vi "Get Message String.vi"(8 "error in (no error)":errorcluster, 11 "SECS-II Class in":refnum<class "SECS-II Class.lvclass">) -> (0 "error out":errorcluster, 2 "String":string, 3 "SECS-II Class out":refnum<class "SECS-II Class.lvclass">)   [LabVIEW 2020, in "SECS Communication.lvlib" / "SECS-II Class.lvclass"]
uses:
  SECS-II Class.lvclass
  SECS-II Class.lvclass/SECS-II Class.ctl
  Variant To Data_ASCII.vi
  Variant To Data_Character.vi
  Variant To Data_Binary.vi
  Variant To Data_Boolean.vi
  Variant To Data_J.vi
  Variant To Data_I1.vi
  Variant To Data_I2.vi
  Variant To Data_I4.vi
  Variant To Data_I8.vi
  Variant To Data_U1.vi
  Variant To Data_U2.vi
  Variant To Data_U4.vi
  Variant To Data_U8.vi
  Variant To Data_F4.vi
  Variant To Data_F8.vi
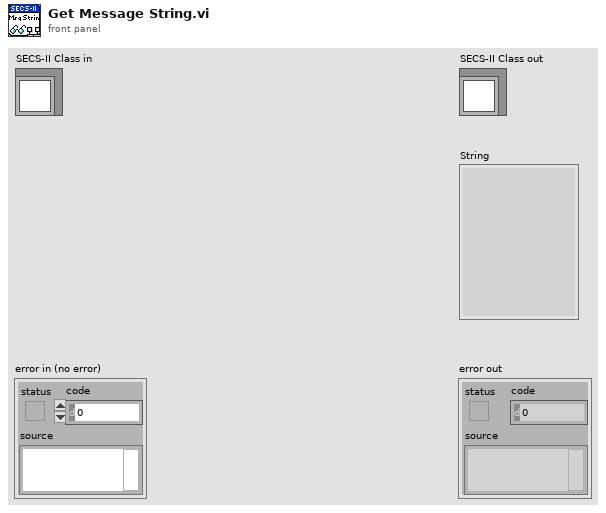
[diagram p1: front panel]
types:
  T1 = typedef "SECS Communication.lvlib/SECS-II Class.lvclass/Message Data.ctl" = cluster{"Index":i32, "Data Item Format":T2, "Format Code":T3, "Parent Index":i32, "Child Index":i32[], "Data":variant}
  T2 = typedef "SECS Communication.lvlib/SECS-II Class.lvclass/Data Item Format.ctl" = enum16{"Data Type", "Value"}
  T3 = typedef "SECS Communication.lvlib/SECS-II Class.lvclass/Format Code.ctl" = enum16{"L", "A", "B", "Boolean", "J", "I1", "I2", "I4", "I8", "U1", "U2", "U4", "U8", "F4", "F8", "Char"}
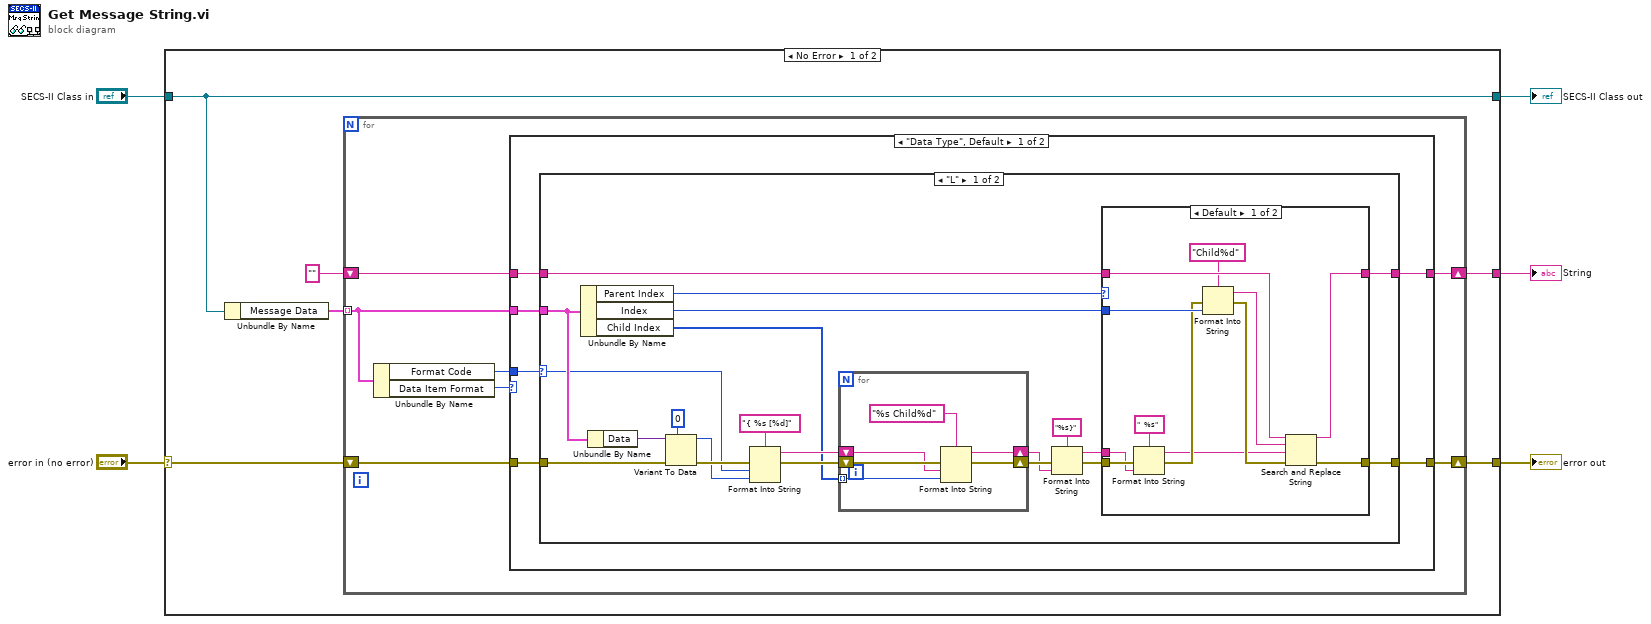
[diagram p0: block diagram]
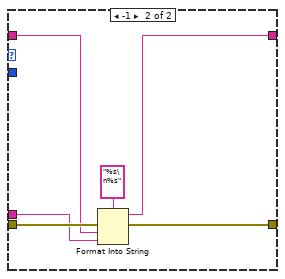
[diagram p2: hidden frame]
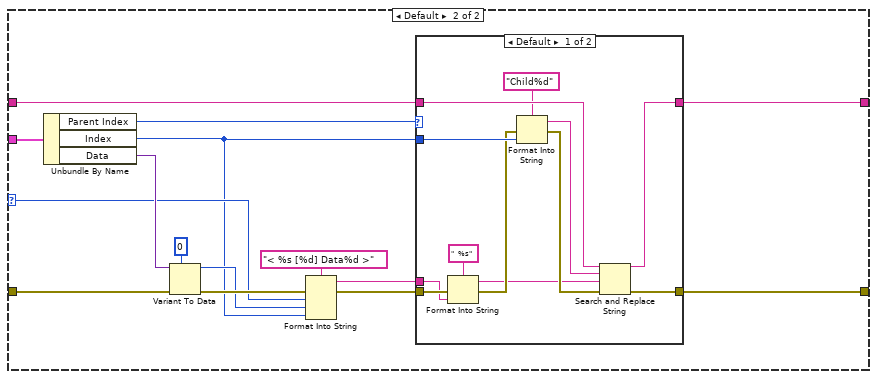
[diagram p3: hidden frame]
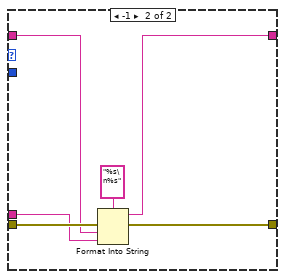
[diagram p4: hidden frame]
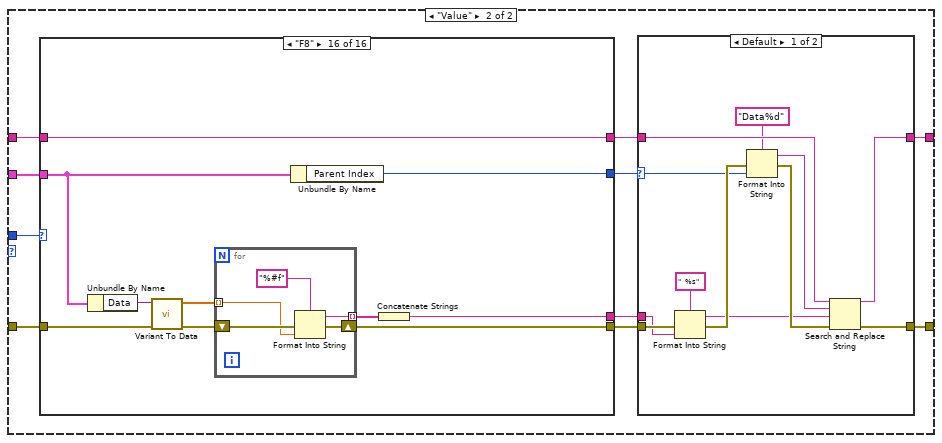
[diagram p5: hidden frame]
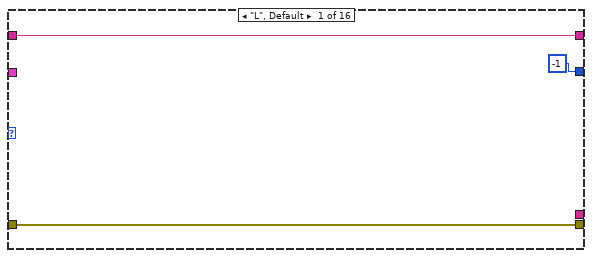
[diagram p7: hidden frame]
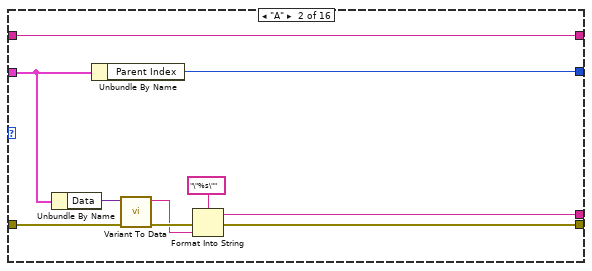
[diagram p8: hidden frame]
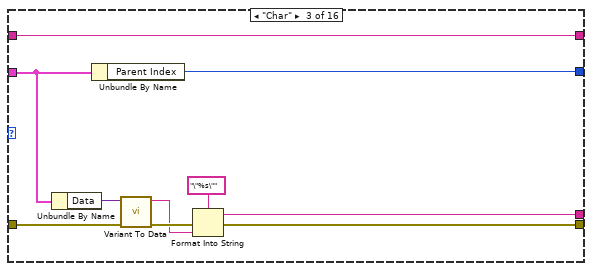
[diagram p9: hidden frame]
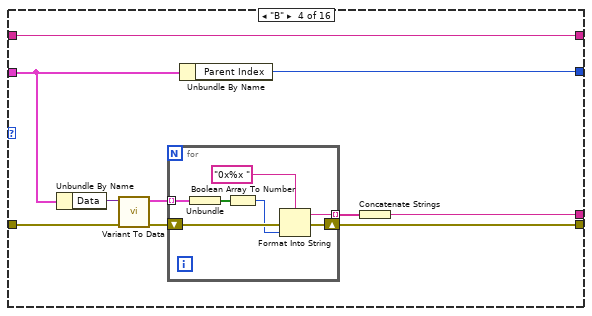
[diagram p10: hidden frame]
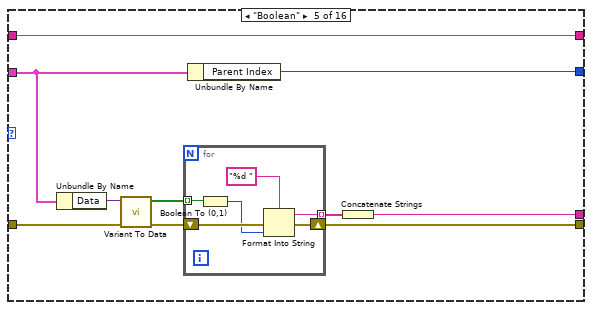
[diagram p11: hidden frame]
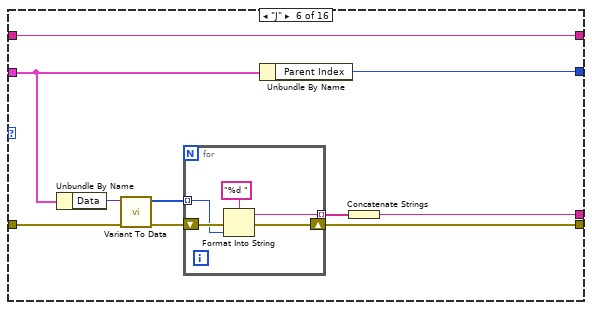
[diagram p12: hidden frame]
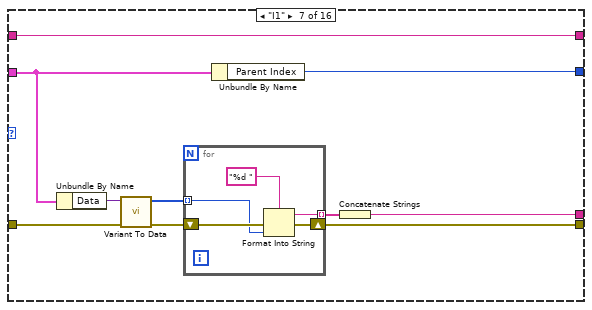
[diagram p13: hidden frame]
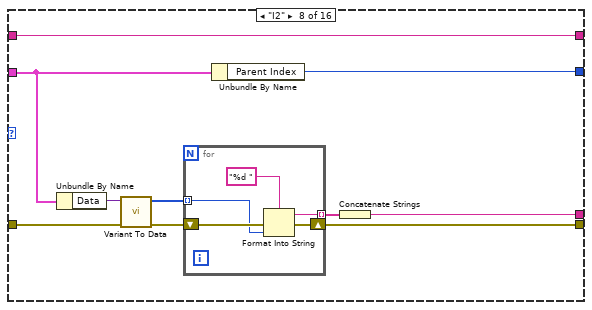
[diagram p14: hidden frame]
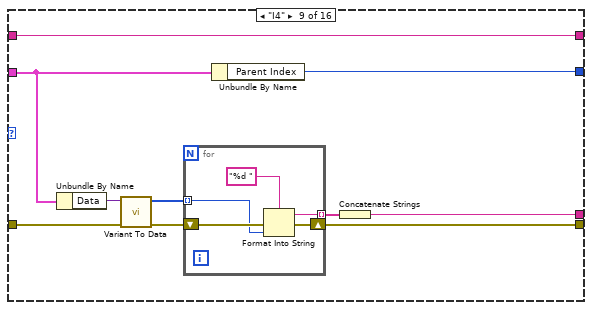
[diagram p15: hidden frame]
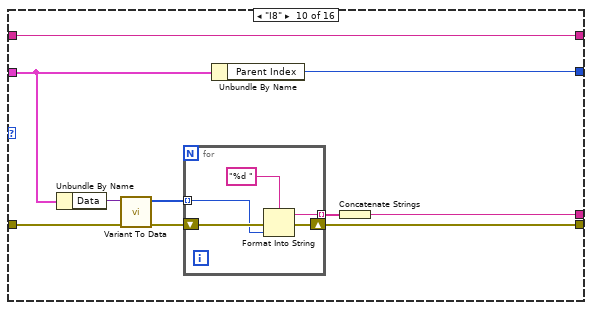
[diagram p16: hidden frame]
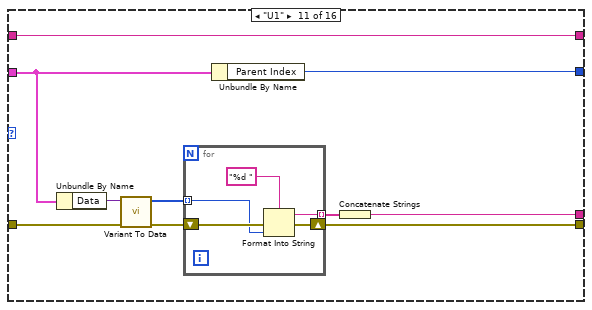
[diagram p17: hidden frame]
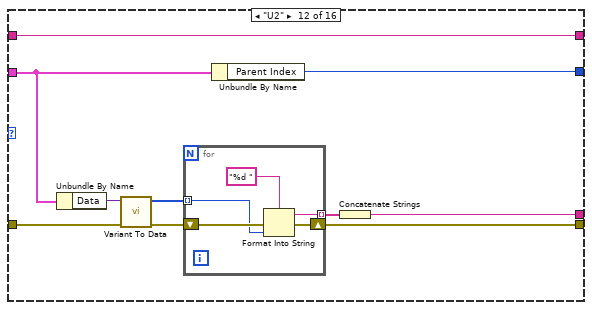
[diagram p18: hidden frame]
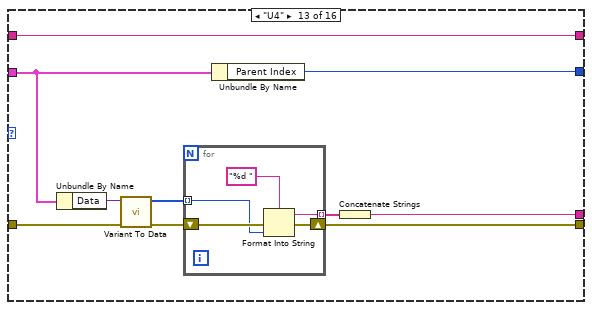
[diagram p19: hidden frame]
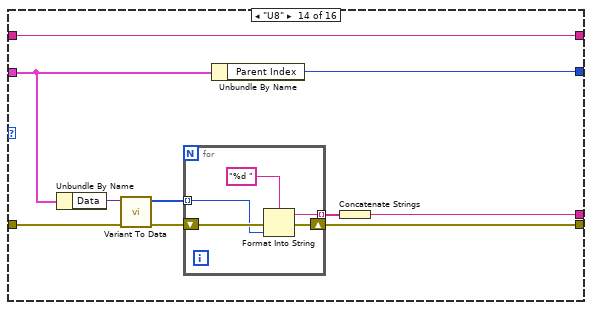
[diagram p20: hidden frame]
diagram:
  n1 = case shown="No Error" "error in (no error)" {
    selector: "error in (no error)" -> [w11 w349]
    tunnel: [w10 w349] -> w5
    tunnel: [w7 w348] -> w4
    tunnel: "SECS-II Class in" -> [w7 w348]
    tunnel: [w6 _] -> w3
    frame No Error {
      n2 = Unbundle By Name(w7) -> ("Message Data"=w8:T1[])
      n3 = for {
        tunnel: w8 -> [w16] mode=indexing
        shift-right: [w12] -> w10
        shift-left: w11 -> [w18]
        shift-right: [w13] -> w6
        shift-left: "" -> [w15]
        n4 = Unbundle By Name(w16) -> ("Format Code"=w14:T3, "Data Item Format"=w17:T2)
        n5 = case shown="\"Data Type\", Default" w17 {
          tunnel: w18 -> [w23 w111]
          tunnel: w16 -> [w22 w109]
          tunnel: w15 -> [w21 w110]
          tunnel: w14 -> [w24 w112]
          tunnel: [w20 w104] -> w13
          tunnel: [w19 w103] -> w12
          frame "Data Type", Default {
            n6 = case shown="\"L\"" w24 {
              selector: w24 -> [w25 w78]
              tunnel: w23 -> [w45 w82]
              tunnel: w22 -> [w37 w84]
              tunnel: w21 -> [w36 w76]
              tunnel: [w34 w71] -> w20
              tunnel: [w33 w70] -> w19
              frame "L" {
                n7 = Unbundle By Name(w37) -> ("Parent Index"=w32:i32, "Index"=w31:i32, "Child Index"=w35:i32[])
                n8 = Unbundle By Name(w37) -> ("Data"=w44:variant)
                n9 = Variant To Data(error in=w45, type=0, Variant=w44) -> (data=w40:i32, error out=w42:errorcluster)
                n10 = Format Into String(format string="{ %s [%d]", error in=w42, w25, w40) -> (resulting string=w38:string, error out=w41:errorcluster)  [unwired: 1 in]
                n11 = for {
                  shift-right: [w67] -> w29
                  shift-left: w38 -> [w68]
                  shift-right: [w66] -> w30
                  shift-left: w41 -> [w69]
                  tunnel: w35 -> [w64] mode=indexing
                  n12 = Format Into String(format string="%s Child%d", error in=w69, w68, w64) -> (resulting string=w67:string, error out=w66:errorcluster)  [unwired: 1 in]
                }
                n13 = Format Into String(format string="%s}", error in=w30, w29) -> (resulting string=w27:string, error out=w28:errorcluster)  [unwired: 1 in]
                n14 = case shown="Default" w32 {
                  tunnel: w28 -> [w50 w63]
                  tunnel: w27 -> [w49 w61]
                  tunnel: w36 -> [w57 w62]
                  tunnel: [w53 w59] -> w34
                  tunnel: [w52 w58] -> w33
                  tunnel: w31 -> [w55 _]
                  frame Default {
                    n15 = Format Into String(format string="  %s", error in=w50, w49) -> (resulting string=w46:string, error out=w48:errorcluster)  [unwired: 1 in]
                    n16 = Format Into String(format string="Child%d", error in=w48, w55) -> (resulting string=w51:string, error out=w54:errorcluster)  [unwired: 1 in]
                    n17 = Search and Replace String(input string=w57, search string=w51, replace string=w46, error in=w54) -> (result string=w53:string, error out=w52:errorcluster)  [unwired: 4 in, 2 out]
                  }
                  frame -1 {
                    n18 = Format Into String(format string="%s\n%s", error in=w63, w62, w61) -> (resulting string=w59:string, error out=w58:errorcluster)  [unwired: 1 in]
                  }
                }
              }
              frame Default {
                n19 = Unbundle By Name(w84) -> ("Parent Index"=w75:i32, "Index"=w72:i32, "Data"=w81:variant)
                n20 = Variant To Data(error in=w82, type=0, Variant=w81) -> (data=w77:i32, error out=w79:errorcluster)
                n21 = Format Into String(format string="< %s [%d] Data%d >", error in=w79, w78, w77, w72) -> (resulting string=w73:string, error out=w74:errorcluster)  [unwired: 1 in]
                n22 = case shown="Default" w75 {
                  tunnel: w74 -> [w89 w102]
                  tunnel: w73 -> [w88 w100]
                  tunnel: w76 -> [w96 w101]
                  tunnel: [w92 w98] -> w71
                  tunnel: [w91 w97] -> w70
                  tunnel: w72 -> [w94 _]
                  frame Default {
                    n23 = Format Into String(format string="  %s", error in=w89, w88) -> (resulting string=w85:string, error out=w87:errorcluster)  [unwired: 1 in]
                    n24 = Format Into String(format string="Child%d", error in=w87, w94) -> (resulting string=w90:string, error out=w93:errorcluster)  [unwired: 1 in]
                    n25 = Search and Replace String(input string=w96, search string=w90, replace string=w85, error in=w93) -> (result string=w92:string, error out=w91:errorcluster)  [unwired: 4 in, 2 out]
                  }
                  frame -1 {
                    n26 = Format Into String(format string="%s\n%s", error in=w102, w101, w100) -> (resulting string=w98:string, error out=w97:errorcluster)  [unwired: 1 in]
                  }
                }
              }
            }
          }
          frame "Value" {
            n27 = case shown="\"F8\"" w112 {
              tunnel: w111 -> [w128 w137 w147 w158 w175 w191 w206 w221 w236 w251 w266 w281 w296 w311 w326 w341]
              tunnel: w110 -> [w129 w134 w144 w153 w169 w185 w200 w215 w230 w245 w260 w275 w290 w305 w320 w335]
              tunnel: [w129 w134 w144 w153 w169 w185 w200 w215 w230 w245 w260 w275 w290 w305 w320 w335] -> w105
              tunnel: w109 -> [_ w135 w145 w157 w174 w190 w205 w220 w235 w250 w265 w280 w295 w310 w325 w340]
              tunnel: [w128 w131 w141 w151 w168 w184 w199 w214 w229 w244 w259 w274 w289 w304 w319 w334] -> w108
              tunnel: [_ w132 w142 w150 w167 w183 w198 w213 w228 w243 w258 w273 w288 w303 w318 w333] -> w107
              tunnel: [-1 ("Parent Index") w133 w143 w152 w170 w186 w201 w216 w231 w246 w261 w276 w291 w306 w321 w336] -> w106
              frame "L", Default {
              }
              frame "A" {
                n28 = Unbundle By Name(w135) -> ("Data"=w139:variant)
                n29 = Unbundle By Name(w135) -> ("Parent Index"=w133:i32)
                n30 = call-poly "Variant To Data.vi"("error in (no error)"=w137, "Variant"=w139) -> ("error out"=w136:errorcluster, "Data"=w130:string)  [unwired: 7 in, 1 out]
                n31 = Format Into String(format string="\"%s\"", error in=w136, w130) -> (resulting string=w132:string, error out=w131:errorcluster)  [unwired: 1 in]
              }
              frame "Char" {
                n32 = Unbundle By Name(w145) -> ("Data"=w149:variant)
                n33 = Unbundle By Name(w145) -> ("Parent Index"=w143:i32)
                n34 = call-poly "Variant To Data.vi"("error in (no error)"=w147, "Variant"=w149) -> ("error out"=w146:errorcluster, "Data"=w140:string)  [unwired: 7 in, 1 out]
                n35 = Format Into String(format string="\"%s\"", error in=w146, w140) -> (resulting string=w142:string, error out=w141:errorcluster)  [unwired: 1 in]
              }
              frame "B" {
                n36 = Unbundle By Name(w157) -> ("Data"=w159:variant)
                n37 = call-poly "Variant To Data.vi"("error in (no error)"=w158, "Variant"=w159) -> ("error out"=w156:errorcluster, "Data Cluster"=w155:cluster{"Data":bool[]}[])  [unwired: 7 in, 1 out]
                n38 = for {
                  tunnel: w155 -> [w165] mode=indexing
                  shift-right: [w161] -> w151
                  shift-left: w156 -> [w164]
                  tunnel: [w160] -> w154 mode=indexing
                  n39 = Unbundle(w165) -> ("Data"=w166:bool[])
                  n40 = Boolean Array To Number(Boolean array=w166) -> (number=w163:u32)
                  n41 = Format Into String(format string="0x%x ", error in=w164, w163) -> (resulting string=w160:string, error out=w161:errorcluster)  [unwired: 1 in]
                }
                n42 = Unbundle By Name(w157) -> ("Parent Index"=w152:i32)
                n43 = Concatenate Strings(w154) -> (w150:string)
              }
              frame "Boolean" {
                n44 = Unbundle By Name(w174) -> ("Data"=w176:variant)
                n45 = call-poly "Variant To Data.vi"("error in (no error)"=w175, "Variant"=w176) -> ("error out"=w173:errorcluster, "Data"=w172:bool[])  [unwired: 7 in, 1 out]
                n46 = for {
                  tunnel: w172 -> [w179] mode=indexing
                  shift-right: [w181] -> w168
                  shift-left: w173 -> [w182]
                  tunnel: [w180] -> w171 mode=indexing
                  n47 = Boolean To (0,1)(Boolean=w179) -> (0, 1=w178:i16)
                  n48 = Format Into String(format string="%d ", error in=w182, w178) -> (resulting string=w180:string, error out=w181:errorcluster)  [unwired: 1 in]
                }
                n49 = Unbundle By Name(w174) -> ("Parent Index"=w170:i32)
                n50 = Concatenate Strings(w171) -> (w167:string)
              }
              frame "J" {
                n51 = Unbundle By Name(w190) -> ("Data"=w192:variant)
                n52 = call-poly "Variant To Data.vi"("error in (no error)"=w191, "Variant"=w192) -> ("error out"=w189:errorcluster, "Data"=w188:i64[])  [unwired: 7 in, 1 out]
                n53 = for {
                  tunnel: w188 -> [w193] mode=indexing
                  shift-right: [w196] -> w184
                  shift-left: w189 -> [w197]
                  tunnel: [w195] -> w187 mode=indexing
                  n54 = Format Into String(format string="%d ", error in=w197, w193) -> (resulting string=w195:string, error out=w196:errorcluster)  [unwired: 1 in]
                }
                n55 = Unbundle By Name(w190) -> ("Parent Index"=w186:i32)
                n56 = Concatenate Strings(w187) -> (w183:string)
              }
              frame "I1" {
                n57 = Unbundle By Name(w205) -> ("Data"=w207:variant)
                n58 = call-poly "Variant To Data.vi"("error in (no error)"=w206, "Variant"=w207) -> ("error out"=w204:errorcluster, "Data"=w203:i8[])  [unwired: 7 in, 1 out]
                n59 = for {
                  tunnel: w203 -> [w208] mode=indexing
                  shift-right: [w211] -> w199
                  shift-left: w204 -> [w212]
                  tunnel: [w210] -> w202 mode=indexing
                  n60 = Format Into String(format string="%d ", error in=w212, w208) -> (resulting string=w210:string, error out=w211:errorcluster)  [unwired: 1 in]
                }
                n61 = Unbundle By Name(w205) -> ("Parent Index"=w201:i32)
                n62 = Concatenate Strings(w202) -> (w198:string)
              }
              frame "I2" {
                n63 = Unbundle By Name(w220) -> ("Data"=w222:variant)
                n64 = call-poly "Variant To Data.vi"("error in (no error)"=w221, "Variant"=w222) -> ("error out"=w219:errorcluster, "Data"=w218:i16[])  [unwired: 7 in, 1 out]
                n65 = for {
                  tunnel: w218 -> [w223] mode=indexing
                  shift-right: [w226] -> w214
                  shift-left: w219 -> [w227]
                  tunnel: [w225] -> w217 mode=indexing
                  n66 = Format Into String(format string="%d ", error in=w227, w223) -> (resulting string=w225:string, error out=w226:errorcluster)  [unwired: 1 in]
                }
                n67 = Unbundle By Name(w220) -> ("Parent Index"=w216:i32)
                n68 = Concatenate Strings(w217) -> (w213:string)
              }
              frame "I4" {
                n69 = Unbundle By Name(w235) -> ("Data"=w237:variant)
                n70 = call-poly "Variant To Data.vi"("error in (no error)"=w236, "Variant"=w237) -> ("error out"=w234:errorcluster, "Data"=w233:i32[])  [unwired: 7 in, 1 out]
                n71 = for {
                  tunnel: w233 -> [w238] mode=indexing
                  shift-right: [w241] -> w229
                  shift-left: w234 -> [w242]
                  tunnel: [w240] -> w232 mode=indexing
                  n72 = Format Into String(format string="%d ", error in=w242, w238) -> (resulting string=w240:string, error out=w241:errorcluster)  [unwired: 1 in]
                }
                n73 = Unbundle By Name(w235) -> ("Parent Index"=w231:i32)
                n74 = Concatenate Strings(w232) -> (w228:string)
              }
              frame "I8" {
                n75 = Unbundle By Name(w250) -> ("Data"=w252:variant)
                n76 = call-poly "Variant To Data.vi"("error in (no error)"=w251, "Variant"=w252) -> ("error out"=w249:errorcluster, "Data"=w248:i64[])  [unwired: 7 in, 1 out]
                n77 = for {
                  tunnel: w248 -> [w253] mode=indexing
                  shift-right: [w256] -> w244
                  shift-left: w249 -> [w257]
                  tunnel: [w255] -> w247 mode=indexing
                  n78 = Format Into String(format string="%d ", error in=w257, w253) -> (resulting string=w255:string, error out=w256:errorcluster)  [unwired: 1 in]
                }
                n79 = Unbundle By Name(w250) -> ("Parent Index"=w246:i32)
                n80 = Concatenate Strings(w247) -> (w243:string)
              }
              frame "U1" {
                n81 = Unbundle By Name(w265) -> ("Data"=w267:variant)
                n82 = call-poly "Variant To Data.vi"("error in (no error)"=w266, "Variant"=w267) -> ("error out"=w264:errorcluster, "Data"=w263:u8[])  [unwired: 7 in, 1 out]
                n83 = for {
                  tunnel: w263 -> [w268] mode=indexing
                  shift-right: [w271] -> w259
                  shift-left: w264 -> [w272]
                  tunnel: [w270] -> w262 mode=indexing
                  n84 = Format Into String(format string="%d ", error in=w272, w268) -> (resulting string=w270:string, error out=w271:errorcluster)  [unwired: 1 in]
                }
                n85 = Unbundle By Name(w265) -> ("Parent Index"=w261:i32)
                n86 = Concatenate Strings(w262) -> (w258:string)
              }
              frame "U2" {
                n87 = Unbundle By Name(w280) -> ("Data"=w282:variant)
                n88 = call-poly "Variant To Data.vi"("error in (no error)"=w281, "Variant"=w282) -> ("error out"=w279:errorcluster, "Data"=w278:u16[])  [unwired: 7 in, 1 out]
                n89 = for {
                  tunnel: w278 -> [w283] mode=indexing
                  shift-right: [w286] -> w274
                  shift-left: w279 -> [w287]
                  tunnel: [w285] -> w277 mode=indexing
                  n90 = Format Into String(format string="%d ", error in=w287, w283) -> (resulting string=w285:string, error out=w286:errorcluster)  [unwired: 1 in]
                }
                n91 = Unbundle By Name(w280) -> ("Parent Index"=w276:i32)
                n92 = Concatenate Strings(w277) -> (w273:string)
              }
              frame "U4" {
                n93 = Unbundle By Name(w295) -> ("Data"=w297:variant)
                n94 = call-poly "Variant To Data.vi"("error in (no error)"=w296, "Variant"=w297) -> ("error out"=w294:errorcluster, "Data"=w293:u32[])  [unwired: 7 in, 1 out]
                n95 = for {
                  tunnel: w293 -> [w298] mode=indexing
                  shift-right: [w301] -> w289
                  shift-left: w294 -> [w302]
                  tunnel: [w300] -> w292 mode=indexing
                  n96 = Format Into String(format string="%d ", error in=w302, w298) -> (resulting string=w300:string, error out=w301:errorcluster)  [unwired: 1 in]
                }
                n97 = Unbundle By Name(w295) -> ("Parent Index"=w291:i32)
                n98 = Concatenate Strings(w292) -> (w288:string)
              }
              frame "U8" {
                n99 = Unbundle By Name(w310) -> ("Data"=w312:variant)
                n100 = call-poly "Variant To Data.vi"("error in (no error)"=w311, "Variant"=w312) -> ("error out"=w309:errorcluster, "Data"=w308:u64[])  [unwired: 7 in, 1 out]
                n101 = for {
                  tunnel: w308 -> [w313] mode=indexing
                  shift-right: [w316] -> w304
                  shift-left: w309 -> [w317]
                  tunnel: [w315] -> w307 mode=indexing
                  n102 = Format Into String(format string="%d ", error in=w317, w313) -> (resulting string=w315:string, error out=w316:errorcluster)  [unwired: 1 in]
                }
                n103 = Unbundle By Name(w310) -> ("Parent Index"=w306:i32)
                n104 = Concatenate Strings(w307) -> (w303:string)
              }
              frame "F4" {
                n105 = Unbundle By Name(w325) -> ("Data"=w327:variant)
                n106 = call-poly "Variant To Data.vi"("error in (no error)"=w326, "Variant"=w327) -> ("error out"=w324:errorcluster, "Data"=w323:sgl[])  [unwired: 7 in, 1 out]
                n107 = for {
                  tunnel: w323 -> [w328] mode=indexing
                  shift-right: [w331] -> w319
                  shift-left: w324 -> [w332]
                  tunnel: [w330] -> w322 mode=indexing
                  n108 = Format Into String(format string="%#f", error in=w332, w328) -> (resulting string=w330:string, error out=w331:errorcluster)  [unwired: 1 in]
                }
                n109 = Unbundle By Name(w325) -> ("Parent Index"=w321:i32)
                n110 = Concatenate Strings(w322) -> (w318:string)
              }
              frame "F8" {
                n111 = Unbundle By Name(w340) -> ("Data"=w342:variant)
                n112 = call-poly "Variant To Data.vi"("error in (no error)"=w341, "Variant"=w342) -> ("error out"=w339:errorcluster, "Data"=w338:dbl[])  [unwired: 7 in, 1 out]
                n113 = for {
                  tunnel: w338 -> [w343] mode=indexing
                  shift-right: [w346] -> w334
                  shift-left: w339 -> [w347]
                  tunnel: [w345] -> w337 mode=indexing
                  n114 = Format Into String(format string="%#f", error in=w347, w343) -> (resulting string=w345:string, error out=w346:errorcluster)  [unwired: 1 in]
                }
                n115 = Unbundle By Name(w340) -> ("Parent Index"=w336:i32)
                n116 = Concatenate Strings(w337) -> (w333:string)
              }
            }
            n117 = case shown="Default" w106 {
              selector: w106 -> [w113 _]
              tunnel: w108 -> [w117 w126]
              tunnel: w107 -> [w116 _]
              tunnel: w105 -> [w124 w125]
              tunnel: [w121 w125] -> w104
              tunnel: [w120 w126] -> w103
              frame Default {
                n118 = Format Into String(format string="  %s", error in=w117, w116) -> (resulting string=w114:string, error out=w115:errorcluster)  [unwired: 1 in]
                n119 = Format Into String(format string="Data%d", error in=w115, w113) -> (resulting string=w119:string, error out=w122:errorcluster)  [unwired: 1 in]
                n120 = Search and Replace String(input string=w124, search string=w119, replace string=w114, error in=w122) -> (result string=w121:string, error out=w120:errorcluster)  [unwired: 4 in, 2 out]
              }
              frame -1 {
              }
            }
          }
        }
      }
    }
    frame Error {
    }
  }
  "error out" <- w5
  "SECS-II Class out" <- w4
  "String" <- w3
